vi "MatlabWriteTimeTest.vi"() -> ()   [LabVIEW 2017]
panel:
  out "Write size":i32
  out "Singles":i32(listbox)
  out "Totals":i32(listbox)
  out "Write":timestamp
  out "Generate Matrix":timestamp
  out "Start":timestamp
  in  "MatrixSIze":i32=1000
  in  "# iterations":i32=100
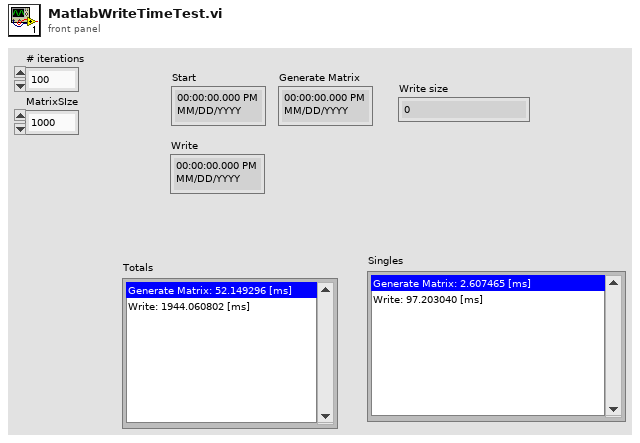
[diagram p1: front panel]
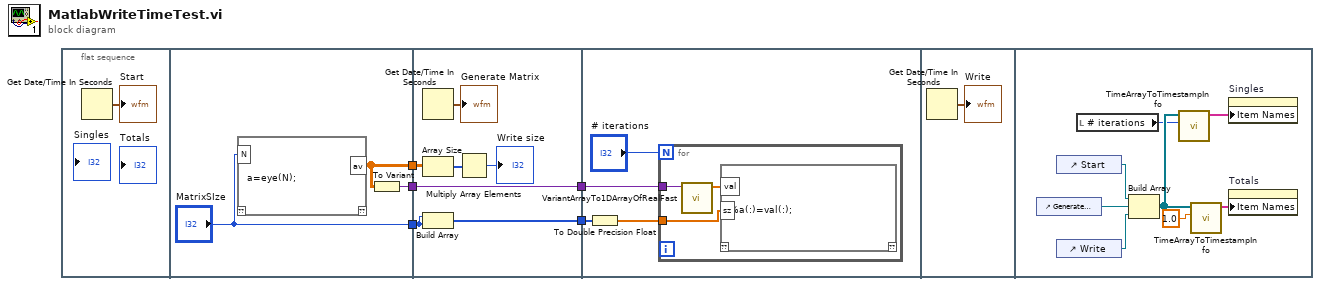
[diagram p0: block diagram]
diagram:
  n1 = flat-sequence {
    tunnel: ["MatrixSIze"] -> w5
    tunnel: [w8] -> w3
    tunnel: [w7] -> w1
    tunnel: w5 -> [w15]
    tunnel: [w14] -> w4
    tunnel: w3 -> [w13]
    tunnel: [w13] -> w2
    tunnel: w1 -> [w12]
    tunnel: w4 -> [w18]
    tunnel: w2 -> [w19]
    frame #0 {
      n2 = Get Date/Time In Seconds() -> (seconds since 1Jan1904=→"Start":timestamp)
    }
    frame #1 {
      n3 = script code="a=eye(N);"("N"="MatrixSIze") -> ("av"=w7:dbl[][])  [unwired: 1 in, 1 out]
      n4 = To Variant(anything=w7) -> (Variant=w8:variant)
    }
    frame #2 {
      n5 = Get Date/Time In Seconds() -> (seconds since 1Jan1904=→"Generate Matrix":timestamp)
      n6 = Array Size(array=w12) -> (size(s)=w10:i32[])
      n7 = Build Array(w15, w15) -> (w14:i32[])
      n8 = Multiply Array Elements(1:w10) -> (0:→"Write size":i32)
    }
    frame #3 {
      n9 = To Double Precision Float(number=w18) -> (double precision float=w17:dbl[])
      n10 = for {
        N: "# iterations" -> [_]
        tunnel: w19 -> [w21]
        tunnel: w17 -> [w23]
        n11 = call "VariantArrayTo1DArrayOfRealFast.vi"("Variant Real Array"=w21) -> ("1D Array"=w22:dbl[])  [unwired: 8 in, 2 out]
        n12 = script code="%a(:)=val(:);"("val"=w22, "sz"=w23) -> ()  [unwired: 1 in, 1 out]
      }
    }
    frame #4 {
      n13 = Get Date/Time In Seconds() -> (seconds since 1Jan1904=→"Write":timestamp)
    }
    frame #5 {
      n14 = control-ref of="Generate Matrix"() -> (w31:refnum<vi>)
      n15 = control-ref of="Start"() -> (w32:refnum<vi>)
      n16 = control-ref of="Write"() -> (w30:refnum<vi>)
      n17 = local read "# iterations"() -> (w28:i32)
      n18 = Build Array(w32, w31, w30) -> (w29:refnum<vi>[])
      n19 = call "TimeArrayToTimestampInfo.vi"("Number of iterations"=w28, "Times array in"=w29) -> ("Array out"=w25:string[])  [unwired: 9 in]
      n20 = call "TimeArrayToTimestampInfo.vi"("Number of iterations"=1.0 ("Times divider"), "Times array in"=w29) -> ("Array out"=w26:string[])  [unwired: 9 in]
      n21 = property on="Singles" class="LstBox (strict)"("Item Names"=w25) -> ()  [unwired: 2 in, 2 out]
      n22 = property on="Totals" class="LstBox (strict)"("Item Names"=w26) -> ()  [unwired: 2 in, 2 out]
    }
  }
